vi "Clear Range.vi"(8 "error in (no error)":errorcluster, 9 "end position (end of line)":cluster{"row":i8, "column":i8}={"row"=-1, "column"=-1}, 10 "start position":cluster{"row":i8, "column":i8}, 11 "HD44780 in":refnum<class "HD44780.lvclass">) -> (0 "error out":errorcluster, 3 "HD44780 out":refnum<class "HD44780.lvclass">)   [LabVIEW 2017, in "HD44780.lvclass"]
uses:
  HD44780.lvclass
  HD44780.lvclass/HD44780.ctl
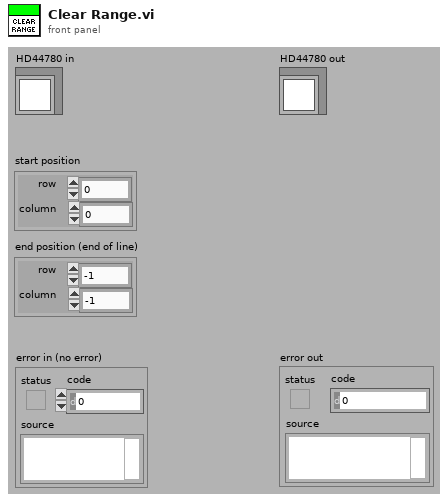
[diagram p1: front panel]
types:
  T1 = typedef "HD44780 Common.lvlib/cluster of class private data.ctl" = cluster{"FPGA VI Reference":refnum<k20>, "device index":i8, "screen size":T2, "font size":T3, "auto wrap":bool, "alignment":T4, "number of line":T5, "shift 0":i8, "entry mode 0":T6, "shift 1":i8, "entry mode 1":T6}
  T2 = typedef "HD44780 Common.lvlib/screen size.ctl" = enum8{"8x1", "8x2", "12x4", "16x1", "16x2", "16x4", "20x1", "20x2", "20x4", "24x1", "24x2", "40x2", "40x4"}
  T3 = typedef "HD44780 Common.lvlib/font size.ctl" = enum8{"5x8", "5x10"}
  T4 = typedef "HD44780 Common.lvlib/alignment.ctl" = enum16{"None", "Left", "Center", "Right"}
  T5 = typedef "HD44780 Common.lvlib/line number.ctl" = enum8{"1 line", "2 lines"}
  T6 = typedef "HD44780 Common.lvlib/entry mode.ctl" = enum8{"increment & no shift", "increment & shift", "decrement & no shift", "decrement & shift"}
  T7 = cluster{"FPGA VI Reference":refnum<k20>, "device index":i8, "screen size":enum8{"8x1", "8x2", "12x4", "16x1", "16x2", "16x4", "20x1", "20x2", "20x4", "24x1", "24x2", "40x2", "40x4"}, "font size":enum8{"5x8", "5x10"}, "auto wrap":bool, "alignment":enum16{"None", "Left", "Center", "Right"}, "number of line":enum8{"1 line", "2 lines"}, "shift 0":i8, "entry mode 0":enum8{"increment & no shift", "increment & shift", "decrement & no shift", "decrement & shift"}, "shift 1":i8, "entry mode 1":enum8{"increment & no shift", "increment & shift", "decrement & no shift", "decrement & shift"}}
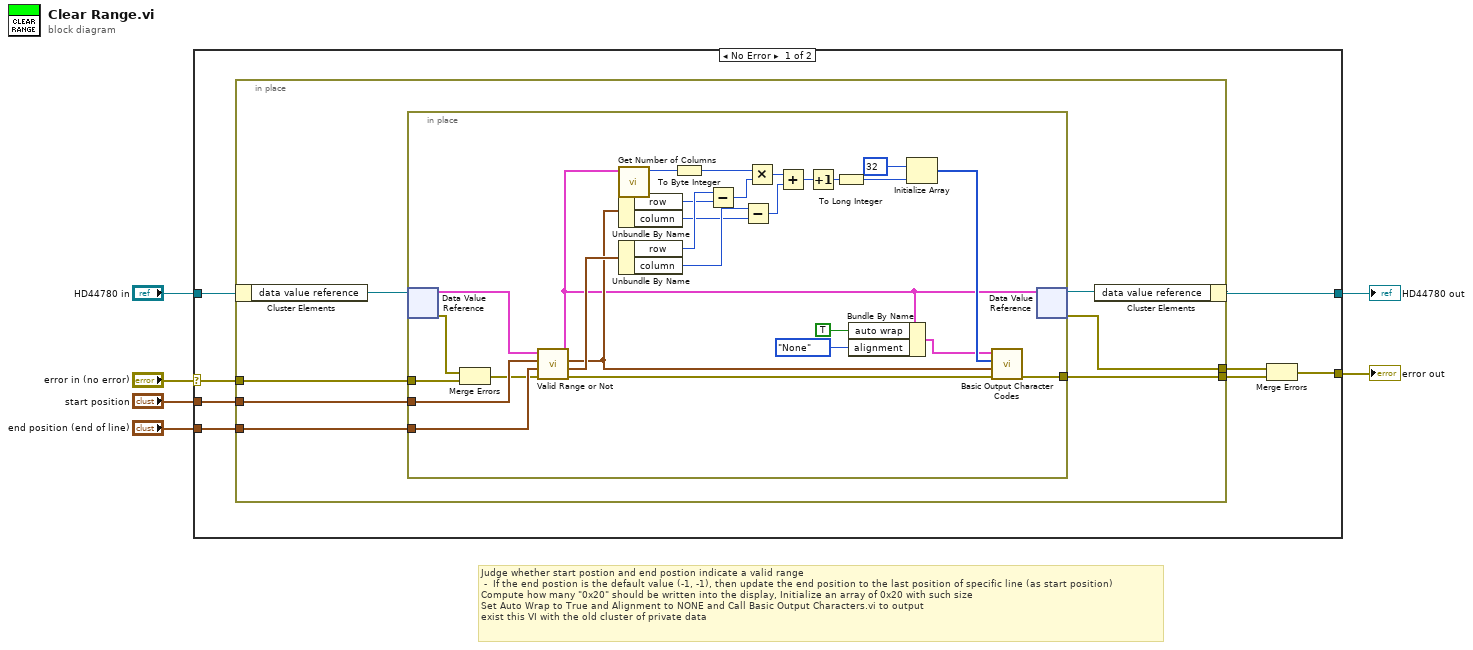
[diagram p0: block diagram]
diagram:
  # "Judge whether start postion and end postion indicate a valid range\n -  If the end postion is the default value (-1, -1), then update the end position to the last position of specific line (as start position)\nCompute how many \"0x20\" should be written into the display, Initialize an array of 0x20 with such size\nSet Auto Wrap to True and Alignment to NONE and Call Basic Output Characters.vi to output\nexist this VI with the old cluster of private data"
  n1 = case shown="No Error" "error in (no error)" {
    selector: "error in (no error)" -> [w12 w51]
    tunnel: "HD44780 in" -> [w11 w50]
    tunnel: "start position" -> [w14 _]
    tunnel: "end position (end of line)" -> [w13 _]
    tunnel: [w7 w51] -> w1
    tunnel: [w10 w50] -> w2
    frame No Error {
      n2 = in-place {
        in-place-border: w14 -> [w21]
        in-place-border: w13 -> [w20]
        in-place-border: w12 -> [w19]
        in-place-border: [w16] -> w9
        in-place-border: [w15] -> w8
        n3 = in-place-cluster #1(w11) -> ("data value reference"=w18:refnum<data-value>)
        n4 = in-place {
          in-place-border: w21 -> [w49]
          in-place-border: w20 -> [w48]
          in-place-border: w19 -> [w47]
          in-place-border: [w29] -> w15
          n5 = in-place-dvr #2(w18) -> (w33:T1, w34:errorcluster)
          n6 = Merge Errors(w34, w47) -> (w35:errorcluster)
          n7 = call "Valid Range or Not.vi"("error in (no error)"=w35, "end position"=w48, "start position"=w49, "cluster of private data in"=w33) -> ("error out"=w30:errorcluster, "end position out"=w46:cluster{"row":i8, "column":i8}, "start position out"=w31:cluster{"row":i8, "column":i8}, "cluster of private data out"=w22:T7)  [unwired: 4 in]
          n8 = call "Get Number of Columns.vi"("cluster of private data in"=w22) -> ("column number"=w43:u8)  [unwired: 10 in]
          n9 = Unbundle By Name(w31) -> ("row"=w44:i8, "column"=w41:i8)
          n10 = Unbundle By Name(w46) -> ("row"=w45:i8, "column"=w42:i8)
          n11 = To Byte Integer(number=w43) -> (8bit integer=w25:i8)
          n12 = Subtract(x=w45, y=w44) -> (x-y=w24:i8)
          n13 = Subtract(x=w42, y=w41) -> (x-y=w23:i8)
          n14 = Multiply(x=w25, y=w24) -> (x*y=w40:i8)
          n15 = Add(x=w40, y=w23) -> (x+y=w38:i8)
          n16 = Increment(x=w38) -> (x+1=w36:i8)
          n17 = To Long Integer(number=w36) -> (32bit integer=w37:i32)
          n18 = Bundle By Name(cluster=w22, "auto wrap"=TRUE, "alignment"=enum16{"None", "Left", "Center", "Right"}."None") -> (w28:T7)
          n19 = Initialize Array(u8 32 ("element"), w37) -> (w32:u8[])
          n20 = call "Basic Output Character Codes.vi"("error in (no error)"=w30, "position (0, 0)"=w31, "character codes"=w32, "cluster of class private data in"=w28) -> ("error out"=w29:errorcluster)  [unwired: 5 in, 2 out]
          n21 = in-place-dvr #2(w22) -> (w17:refnum<data-value>, w16:errorcluster)
        }
        n22 = in-place-cluster #1("data value reference"=w17) -> (w10:refnum<class "HD44780.lvclass">)
      }
      n23 = Merge Errors(w9, w8) -> (w7:errorcluster)
    }
    frame Error {
    }
  }
  "HD44780 out" <- w2
  "error out" <- w1
